vi "Update Report FilePath.vi"(8 "error in (no error)":errorcluster, 11 "Report Path":path) -> (0 "error out":errorcluster)   [LabVIEW 2018]
doc: "This subVI enqueues the named action in to the communications queue along with the input data."
uses:
  Private Controls/Module Action.ctl
  Controller (Host).lvlib
  Private Controls/Module Data.ctl
panel:
  in  "Action":T1=enum."Update Report FilePath"
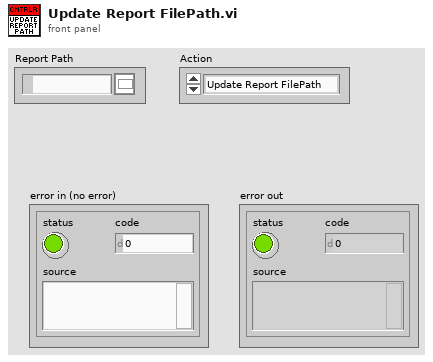
[diagram p1: front panel]
types:
  T1 = typedef "Controller (Host).lvlib/Module Action.ctl" = enum8{"Timeout", "Value to Monitor", "Init", "Reset Dev_Min_Max", "Error", "Exit", "Prompt Test Info", "Prompt Operation Select", "Load APU Setup Data", "Update Report FilePath"}
  T2 = typedef "Controller (Host).lvlib/Module Data.ctl" = cluster{"Data":variant, "Action":T3}
  T3 = typedef "Controller (Host).lvlib/Module Action.ctl" = enum8{"Timeout", "Value to Monitor", "Init", "Reset Dev_Min_Max", "Error", "Exit", "Prompt Test Info", "Prompt Operation Select", "Load APU Setup Data"}
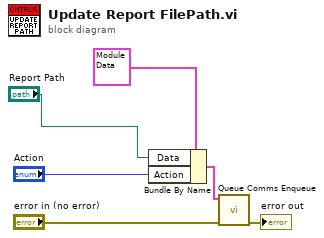
[diagram p0: block diagram]
diagram:
  n1 = Bundle By Name(cluster=T2 {"Data"=variant, "Action"=enum."Init"} ("element"), "Data"="Report Path", "Action"="Action") -> (w6:T2)
  n2 = call "Queue Comms Enqueue.vi"("error in (no error)"="error in (no error)", "element"=w6) -> ("error out"=→"error out":errorcluster)  [unwired: 9 in]
